vi "Add.vi"(5 "Z":dbl, 7 "error in":errorcluster, 8 "Y":dbl, 9 "X":dbl, 10 "Vec3d in":refnum<class "Vec3d.lvclass">) -> (0 "error out":errorcluster, 3 "Vec3d out":refnum<class "Vec3d.lvclass">)   [LabVIEW 2017, in "Vec3d.lvclass"]
uses:
  Vec3d.lvclass
  Vec3d.lvclass/Vec3d.ctl
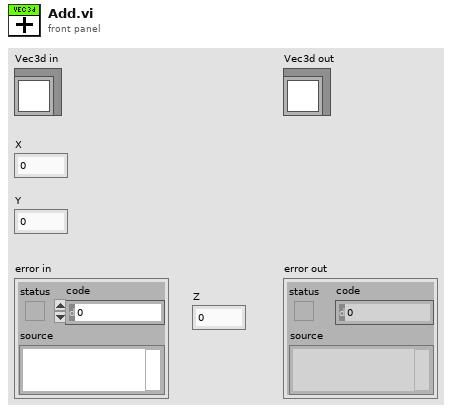
[diagram p1: front panel]
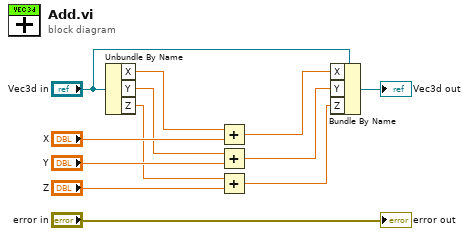
[diagram p0: block diagram]
diagram:
  n1 = Unbundle By Name("Vec3d in") -> ("X"=w8:dbl, "Y"=w7:dbl, "Z"=w6:dbl)
  n2 = Add(x=w8, y="X") -> (x+y=w5:dbl)
  n3 = Add(x=w7, y="Y") -> (x+y=w4:dbl)
  n4 = Add(x=w6, y="Z") -> (x+y=w3:dbl)
  n5 = Bundle By Name(cluster="Vec3d in", "X"=w5, "Y"=w4, "Z"=w3) -> (→"Vec3d out":refnum<class "Vec3d.lvclass">)
  "error out" <- "error in"
